vi "Call Template.vi"(11 "Data In":variant) -> (3 "Data Out":variant)   [LabVIEW 2020]
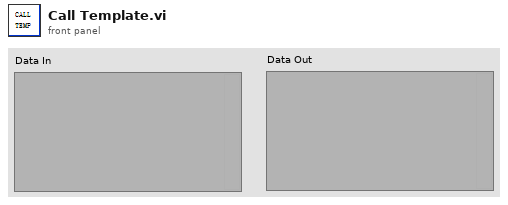
[diagram p1: front panel]
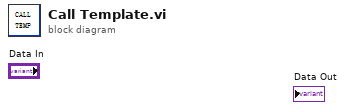
[diagram p0: block diagram]
diagram:
